vi "modcfg serialization.vi"() -> (0 "no error":errorcluster, 3 "name ok":bool)   [LabVIEW 2013, in "TBM Tests.lvlib"]
uses:
  TBM Tests.lvlib
  module configuration/TBM module configuration.lvclass
  <vilib>/NI/Configuration Framework/serializable configuration/NISE_CEF_serializable configuration.lvclass/NISE_CEF_serializable configuration.ctl
  <vilib>/Utility/LVClass/Get LV Class Name.vi
  <vilib>/NI/Configuration Framework/error generator/NISE_error generator.vi
  <vilib>/NI/Configuration Framework/serializable configuration/NISE_CEF_serializable configuration.lvclass
panel:
  out "version":string
  out "data":string
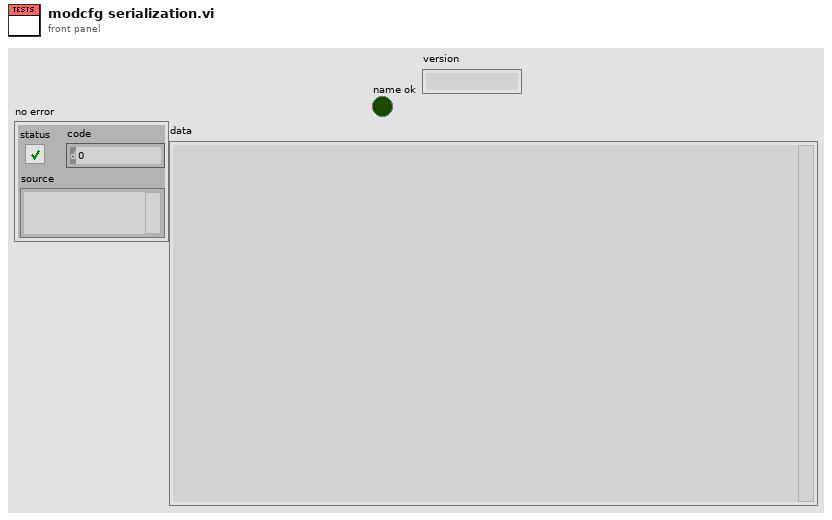
[diagram p1: front panel]
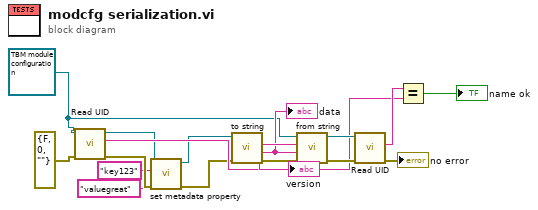
[diagram p0: block diagram]
diagram:
  w9 = refnum<class "TBM module configuration.lvclass"> refnum ("module configuration")
  n1 = call <vilib>:"Read UID.vi"("error in"=errorcluster {"status"=FALSE, "code"=0, "source"=""} ("error out"), "configuration in"=w9) -> ("error out"=w3:errorcluster, "instance id"=w8:string, "configuration out"=w6:refnum<class "TBM module configuration.lvclass">)  [unwired: 7 in]
  n2 = call <vilib>:"set metadata property.vi"("error in"=w3, "value"="valuegreat", "key"="key123", "configuration in"=w6) -> ("error out"=w4:errorcluster, "configuration out"=w5:refnum<class "TBM module configuration.lvclass">)  [unwired: 6 in]
  n3 = call-dynamic "to string.vi"("error in"=w4, "module configuration in"=w5) -> ("error out"=w17:errorcluster, "data"=w11:string, "version"=w16:string)  [unwired: 6 in, 1 out]
  "data" <- w11
  "version" <- w16
  n4 = call-dynamic "from string.vi"("error in"=w17, "data"=w11, "version"=w16, "module configuration in"=w9) -> ("error out"=w14:errorcluster, "module configuration out"=w15:refnum<class "TBM module configuration.lvclass">)  [unwired: 6 in]
  n5 = call <vilib>:"Read UID.vi"("error in"=w14, "configuration in"=w15) -> ("error out"=→"no error":errorcluster, "instance id"=w12:string)  [unwired: 7 in, 1 out]
  n6 = Equal?(x=w12, y=w8) -> (x = y?=→"name ok":bool)
